vi "Channel Subpanel.vi"() -> ()   [LabVIEW 2021, in "CIF Manager UI.lvlib"]
uses:
  CIF Manager UI.lvlib
  CIFUI/Typedef/Channel Connection.ctl
  CIFUI/Typedef/Class Data for SubPanel.ctl
  <vilib>/gRPC/LabVIEW gRPC Library/Shared/grpcId.ctl
  CIFUI/Typedef/Core UI References.ctl
  CIFUI/Typedef/New Plugin.ctl
  CIFUI/Typedef/Run Listen Button.ctl
  CIFUI/Typedef/CIF_Manager_UI_Tab.ctl
  CIFUI/Typedef/SubPanel Events.ctl
  CIFUI/Typedef/New Connection Event Data.ctl
  CIFUI/Typedef/New Connection Plugin Event Data.ctl
  CIFUI/CIF_UI.lvclass
  CIFUI/CIF_UI.lvclass/CIF_UI.ctl
  CIFUI/Typedef/Direction to Include.ctl
  <vilib>/CIF Foundation/CIF Utilities/DataTypes/Typedef/Endian.ctl
  CIFUI/Typedef/Force Channel.ctl
  CIFUI/Utilities/Get Human Readable Error.vi
  <vilib>/CIF Foundation/CIF Utilities/Errors/Append Error Location.vi
  CIFUI/UI Element Update/Empty Tree by Reference.vi
  CIFUI/UI Element Update/Empty Table by Reference.vi
  CIFUI/UI Element Update/Initialize Manager Tab by Reference.vi
  <vilib>/CIF Foundation/CIF Utilities/Errors/Human Readable Error Message.vi
  <vilib>/CIF Foundation/CIF Utilities/DataTypes/DataTypes_CIF_U.lvlib
  <vilib>/gRPC/LabVIEW gRPC Library/grpc-lvsupport-release.lvlib
panel:
  in  "String Force":string
  in  "Class Data for SubPanel":T1
  in  "Force Active":bool
  in  "I64 Force":i64
  in  "U64 Force":u64
  in  "Double Force":dbl
  in  "Forced Data":string
  in  "Channel":string
  in  "Force Channel":bool
  in  "Link Channel":bool
  in  "Connection":T5
  in  "Publisher Channels":string(tree)
  in  "Subscriber Channels":string(tree)
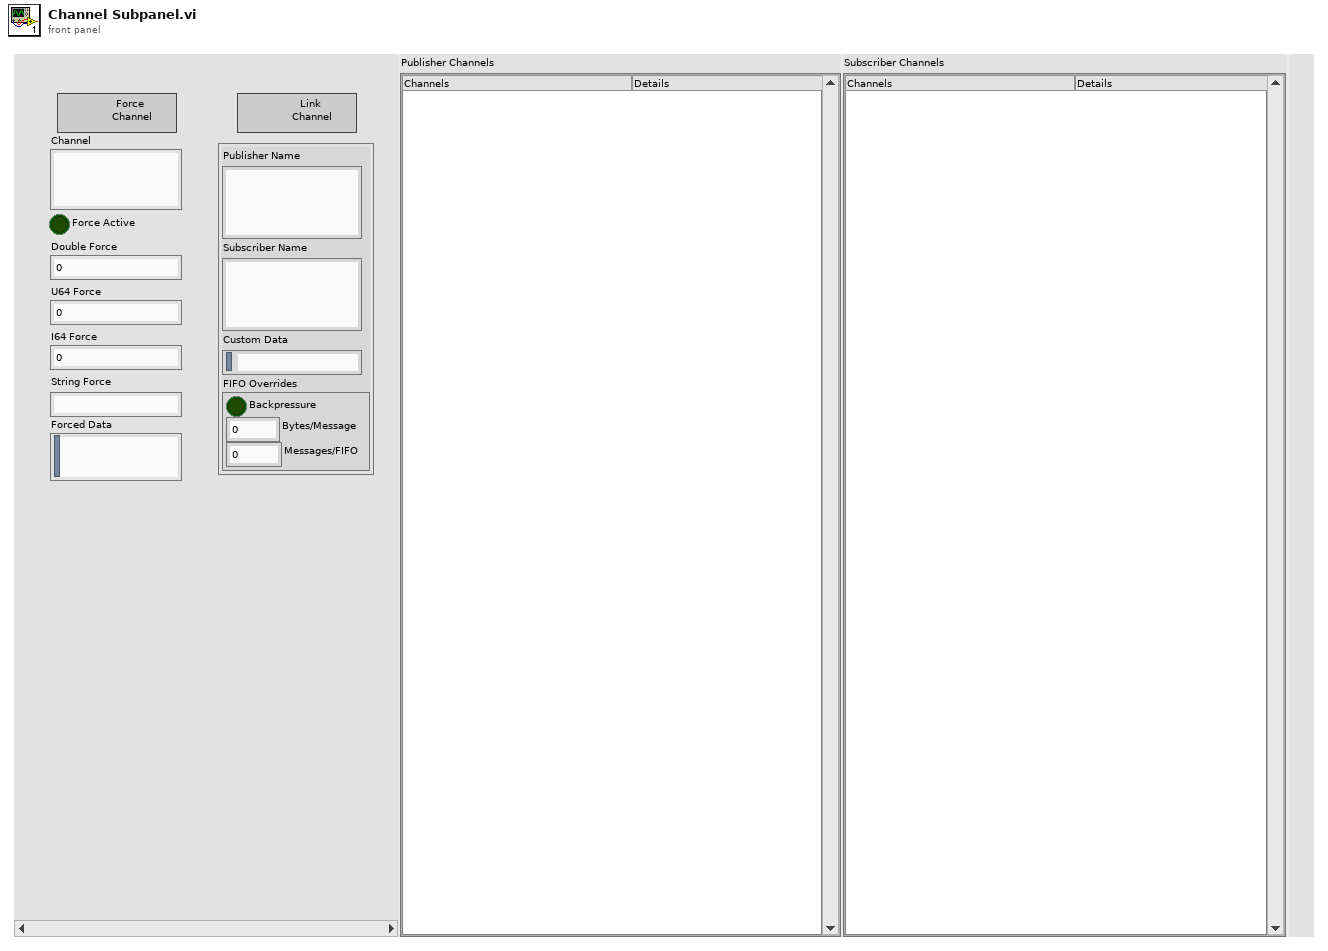
[diagram p1: front panel]
types:
  T1 = typedef "CIF_UI.lvclass/Class Data for SubPanel.ctl" = cluster{"IP Address":string, "Manager gRPC ID":T2, "Server Certificate File (.crt)":path, "Connected":bool, "Manager Connection":bool, "Core UI References":T3, "Subpanel Events":T4}
  T2 = typedef "grpc-lvsupport-release.lvlib/grpcId.ctl" = u64
  T3 = typedef "CIF_UI.lvclass/Core UI References.ctl" = cluster{"Discovered Plugins":refnum<vi>, "Discovered Plugins Valid":bool, "Loaded Plugins":refnum<vi>, "Loaded Plugins Valid":bool, "Publisher Channels":refnum<vi>, "Publisher Channels Valid":bool, "Subscriber Channels":refnum<vi>, "Subscriber Channels Valid":bool, "Plugin Status":refnum<vi>, "Plugin Status Valid":bool, "Channel Connection":refnum<vi>, "Channel Connection Valid":bool, "New Plugin Load":refnum<vi>, "New Plugin Load Valid":bool, "Errors":refnum<vi>, "Errors Valid":bool, "Plugin to Abort":refnum<vi>, "Plugin to Abort Valid":bool, "Connection":refnum<vi>, "Connection Valid":bool, "Exit":refnum<vi>, "Exit Valid":bool, "Run Listen":refnum<vi>, "Run Listen Valid":bool, "CIF Manager Tab":refnum<vi>, "Manger Tab Valid":bool, "Clear Local Error":refnum<vi>, "Clear Local Error Valid":bool, "Local Error":refnum<vi>, "Local Error Valid":bool, "System Errors":refnum<vi>, "System Errors Valid":bool, "Plugin Selection":refnum<vi>, "Plugin Selection Valid":bool}
  T4 = typedef "CIF_UI.lvclass/SubPanel Events.ctl" = cluster{"Clear Local Error":refnum<user-event>, "Shutdown":refnum<user-event>, "gRPC Connection":refnum<user-event>, "Plugin Connection":refnum<user-event>}
  T5 = typedef "CIF_UI.lvclass/Channel Connection.ctl" = cluster{"Publisher Name":string, "Subscriber Name":string, "Custom Data":string, "FIFO Overrides":cluster{"Backpressure":bool, "Bytes/Message":u32, "Messages/FIFO":u32}}
  T6 = typedef "CIF_UI.lvclass/Direction to Include.ctl" = enum16{"All", "Subscriber", "Publisher"}
  T7 = enum16{"big-endian, network order", "native, host order", "little-endian"}
  T8 = typedef "DataTypes_CIF_U.lvlib/Endian.ctl" = enum16{"Little Endian", "Big Endian"}
  T9 = typedef "CIF_UI.lvclass/Force Channel.ctl" = cluster{"channel_name":string, "force":bool, "force_data":string}
  T10 = typedef "CIFCoreChannel_client.lvlib/cif_management_common_Channel.ctl" = cluster{"name":string, "direction":T11, "type":string, "custom_config":u8[], "connected":bool, "connected_name":string, "forced":bool, "channel_pattern":T12}
  T11 = typedef "CIFCoreChannel_client.lvlib/cif_management_common_ChannelDirection.ctl" = enum32{"CHANNELDIRECTION_UNKNOWN", "CHANNELDIRECTION_PUBLISHER", "CHANNELDIRECTION_SUBSCRIBER"}
  T12 = typedef "CIFCoreChannel_client.lvlib/cif_management_common_ChannelPattern.ctl" = enum32{"CHANNELPATTERN_UNKNOWN", "CHANNELPATTERN_TAG", "CHANNELPATTERN_FIFO", "CHANNELPATTERN_MULTIFIFO", "CHANNELPATTERN_BACKPRESSUREFIFO"}
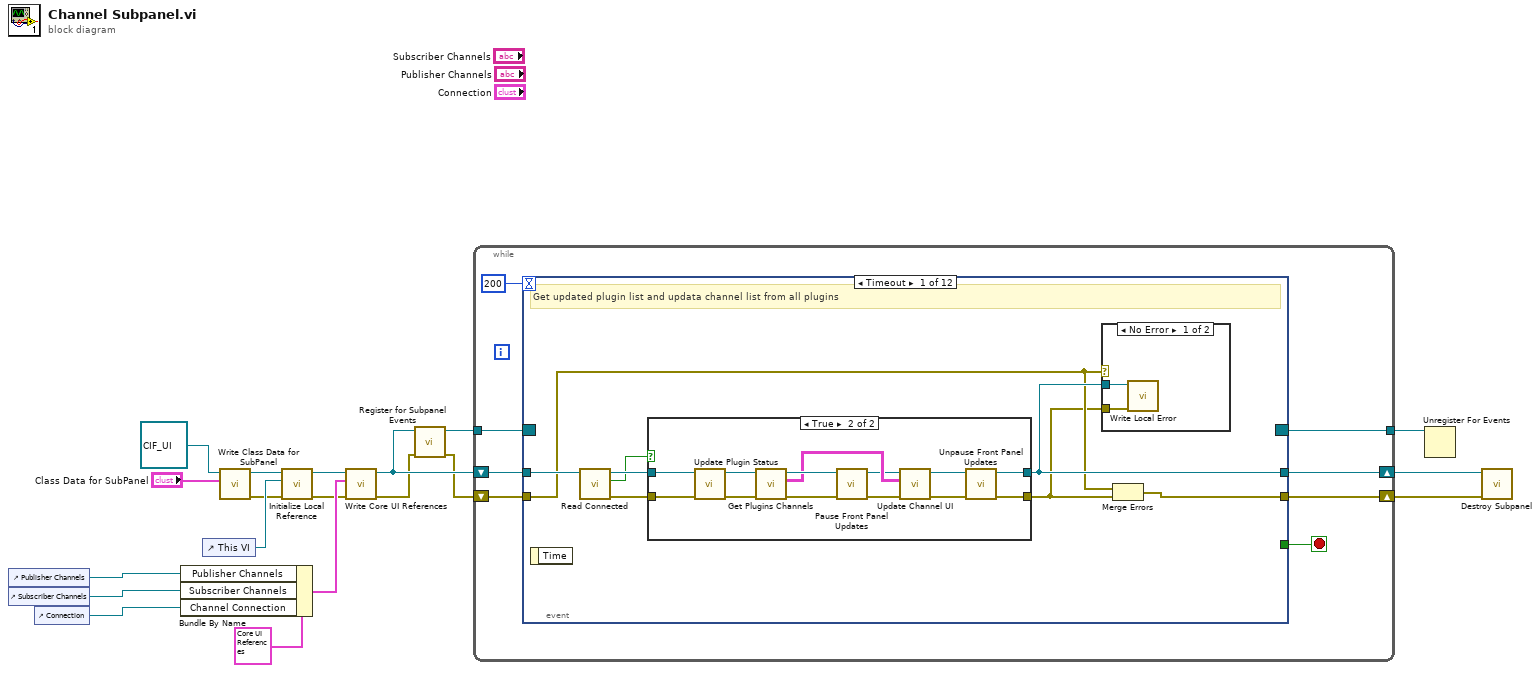
[diagram p0: block diagram]
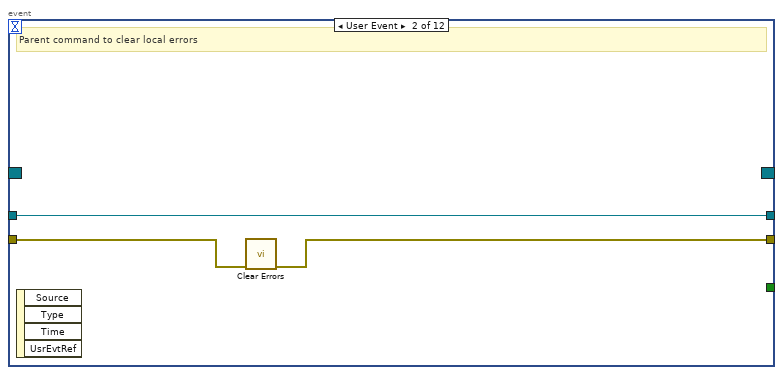
[diagram p4: hidden frame]
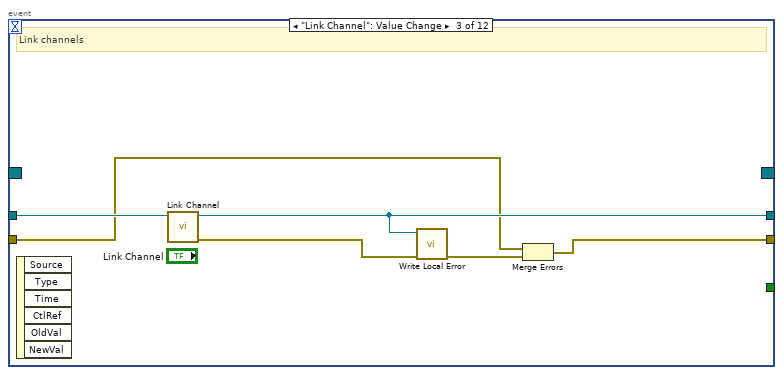
[diagram p5: hidden frame]
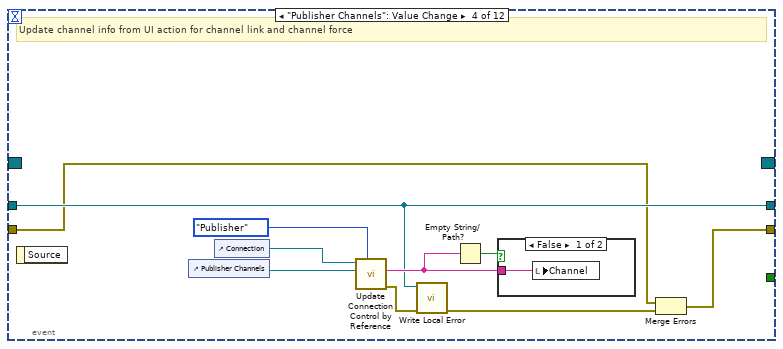
[diagram p6: hidden frame]
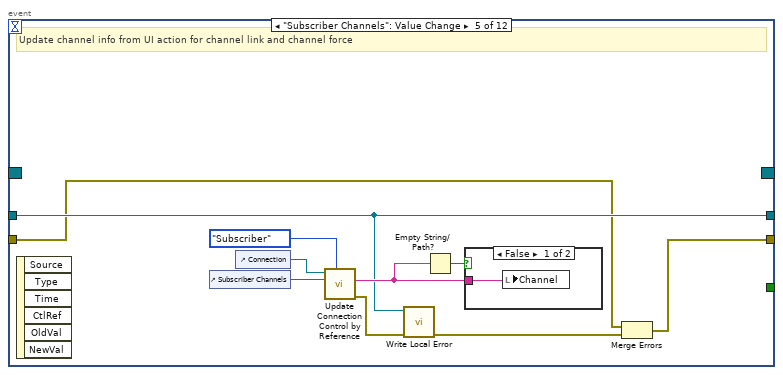
[diagram p8: hidden frame]
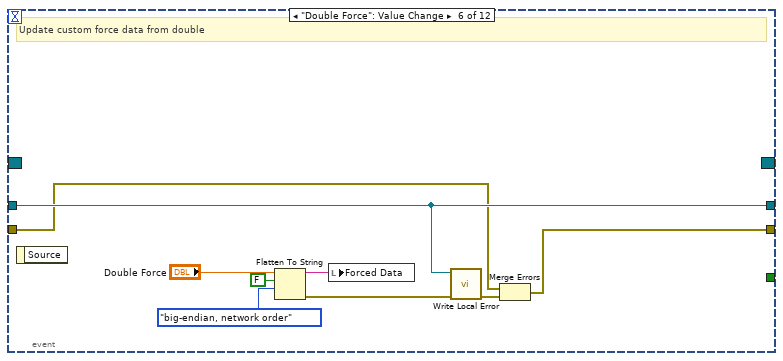
[diagram p10: hidden frame]
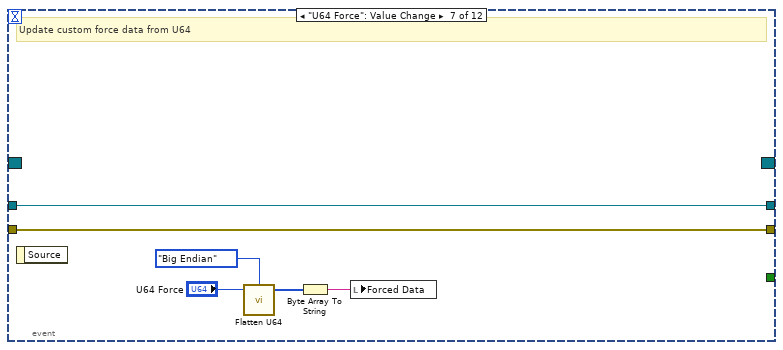
[diagram p11: hidden frame]
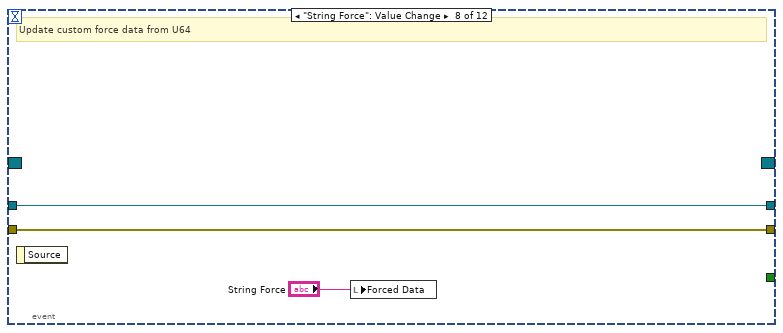
[diagram p12: hidden frame]
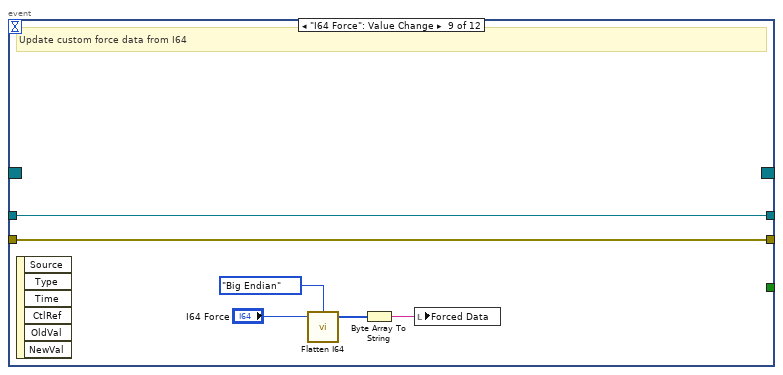
[diagram p13: hidden frame]
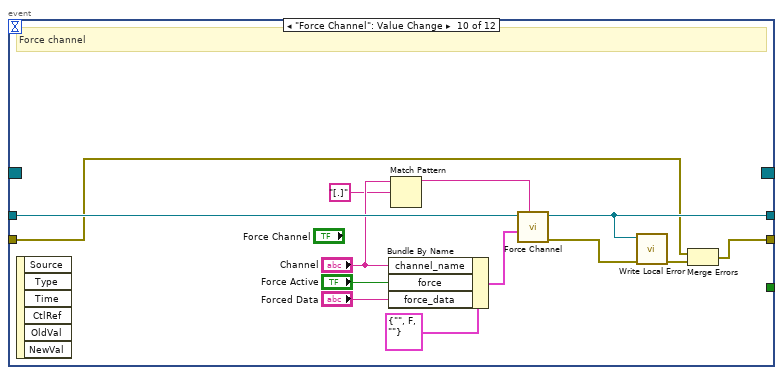
[diagram p14: hidden frame]
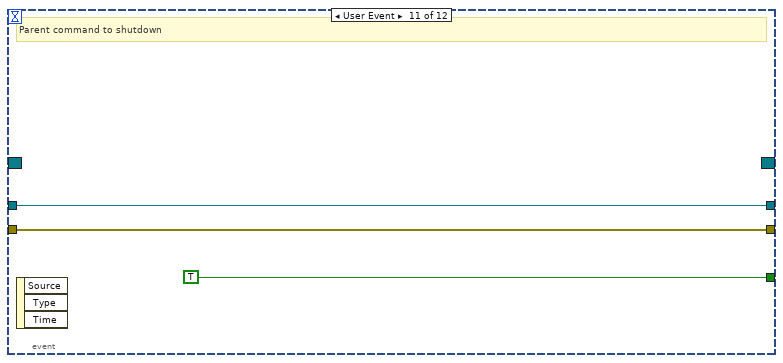
[diagram p15: hidden frame]
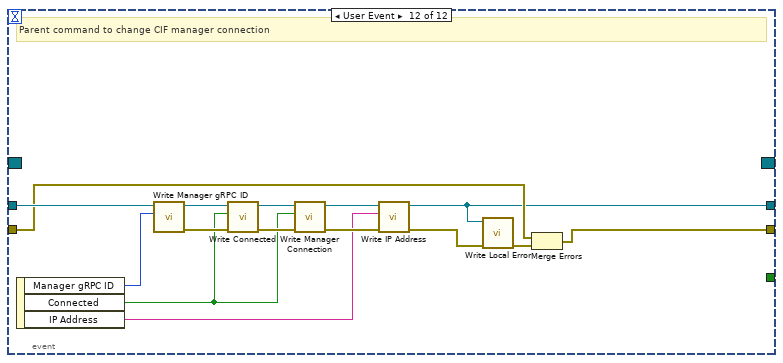
[diagram p16: hidden frame]
diagram:
  n1 = control-ref of="Publisher Channels"() -> (w19:refnum<vi>)
  n2 = control-ref of="Subscriber Channels"() -> (w18:refnum<vi>)
  n3 = control-ref of="Connection"() -> (w17:refnum<vi>)
  n4 = Bundle By Name(cluster=T3 {"Discovered Plugins"=refnum, "Discovered Plugins Valid"=FALSE, "Loaded Plugins"=refnum, "Loaded Plugins Valid"=FALSE, "Publisher Channels"=refnum, "Publisher Channels Valid"=FALSE, "Subscriber Channels"=refnum, "Subscriber Channels Valid"=FALSE, "Plugin Status"=refnum, "Plugin Status Valid"=FALSE, "Channel Connection"=refnum, "Channel Connection Valid"=FALSE, "New Plugin Load"=refnum, "New Plugin Load Valid"=FALSE, "Errors"=refnum, "Errors Valid"=FALSE, "Plugin to Abort"=refnum, "Plugin to Abort Valid"=FALSE, "Connection"=refnum, "Connection Valid"=FALSE, "Exit"=refnum, "Exit Valid"=FALSE, "Run Listen"=refnum, "Run Listen Valid"=FALSE, "CIF Manager Tab"=refnum, "Manger Tab Valid"=FALSE, "Clear Local Error"=refnum, "Clear Local Error Valid"=FALSE, "Local Error"=refnum, "Local Error Valid"=FALSE, "System Errors"=refnum, "System Errors Valid"=FALSE, "Plugin Selection"=refnum, "Plugin Selection Valid"=FALSE} ("UI References"), "Publisher Channels"=w19, "Subscriber Channels"=w18, "Channel Connection"=w17) -> (w15:T3)
  n5 = control-ref of="This VI"() -> (w10:refnum<vi>)
  n6 = call "Write Class Data for SubPanel.vi"("Class Data for SubPanel"="Class Data for SubPanel", "CIF_UI in"=refnum<class "CIF_UI.lvclass"> refnum) -> ("error out"=w3:errorcluster, "CIF_UI out"=w4:refnum<class "CIF_UI.lvclass">)  [unwired: 8 in]
  n7 = call "Initialize Local Reference.vi"("error in (no error)"=w3, "This VI"=w10, "CIF_UI in"=w4) -> ("error out"=w8:errorcluster, "CIF_UI out"=w9:refnum<class "CIF_UI.lvclass">)  [unwired: 7 in]
  n8 = call "Write Core UI References.vi"("error in (no error)"=w8, "UI References"=w15, "CIF_UI in"=w9) -> ("error out"=w12:errorcluster, "CIF_UI out"=w14:refnum<class "CIF_UI.lvclass">)  [unwired: 7 in]
  n9 = call "Register for Subpanel Events.vi"("error in (no error)"=w12, "CIF_UI in"=w14) -> ("error out"=w11:errorcluster, "Event Registration Refnum"=w13:refnum<event-registration>)  [unwired: 8 in]
  n10 = while {
    tunnel: w13 -> [w26]
    shift-right: [w22] -> w7
    shift-left: w14 -> [w24]
    shift-right: [w20] -> w1
    shift-left: w11 -> [w23]
    tunnel: [w21] -> w2
    stop <- w25 stop-if-true
    n11 = event shown="[0] Timeout" {
      selector: w26 -> [_ _ _ _ _ _ _ _ _ _ _ _]
      dyn-events: [_ _ _ _ _ _ _ _ _ _ _ _] -> w21
      timeout: 200 -> [_ _ _ _ _ _ _ _ _ _ _ _]
      tunnel: [_ _ _ _ _ _ _ _ _ _ TRUE _] -> w25
      tunnel: w24 -> [w32 w53 w61 w65 w76 w86 w98 w101 w103 w120 w122 w132]
      tunnel: w23 -> [w30 w55 w57 w63 w73 w85 w97 w100 w102 w108 w121 w125]
      tunnel: [w28 w54 w56 w62 w74 w84 w97 w100 w102 w109 w121 w126] -> w20
      tunnel: [w31 w53 w60 w65 w76 w86 w98 w101 w103 w112 w122 w124] -> w22
      event Timeout {
        # "Get updated plugin list and updata channel list from all plugins"
        n12 = event-data() -> ()  [unwired: 1 in, 1 out]
        n13 = call "Read Connected.vi"("CIF_UI in"=w32) -> ("error out"=w34:errorcluster, "Connected"=w33:bool, "CIF_UI out"=w35:refnum<class "CIF_UI.lvclass">)  [unwired: 8 in]
        n14 = case shown="True" w33 {
          tunnel: w34 -> [w38 w45]
          tunnel: [w38 w52] -> w29
          tunnel: w35 -> [w39 w46]
          tunnel: [w39 w51] -> w31
          frame False {
          }
          frame True {
            n15 = call "Update Plugin Status.vi"("error in (no error)"=w45, "CIF_UI in"=w46) -> ("error out"=w49:errorcluster, "CIF_UI out"=w50:refnum<class "CIF_UI.lvclass">)  [unwired: 8 in]
            n16 = call "Get Plugins Channels.vi"("error in (no error)"=w49, "CIF_UI in"=w50) -> ("error out"=w41:errorcluster, "Channels"=w43:T10[][], "CIF_UI out"=w44:refnum<class "CIF_UI.lvclass">)  [unwired: 6 in, 1 out]
            n17 = call "Pause Front Panel Updates.vi"("error in (no error)"=w41, "CIF_UI in"=w44) -> ("error out"=w40:errorcluster, "CIF_UI out"=w42:refnum<class "CIF_UI.lvclass">)  [unwired: 8 in]
            n18 = call "Update Channel UI.vi"("error in (no error)"=w40, "Channels"=w43, "CIF_UI in"=w42) -> ("error out"=w47:errorcluster, "CIF_UI out"=w48:refnum<class "CIF_UI.lvclass">)  [unwired: 7 in]
            n19 = call "Unpause Front Panel Updates.vi"("error in (no error)"=w47, "CIF_UI in"=w48) -> ("error out"=w52:errorcluster, "CIF_UI out"=w51:refnum<class "CIF_UI.lvclass">)  [unwired: 8 in]
          }
        }
        n20 = case shown="No Error" w30 {
          tunnel: w29 -> [w37 _]
          tunnel: w31 -> [w36 _]
          frame No Error {
            n21 = call "Write Local Error.vi"("error in (no error)"=w37, "CIF_UI in"=w36) -> ()  [unwired: 9 in, 1 out]
          }
          frame Error {
          }
        }
        n22 = Merge Errors(w30, w29) -> (w28:errorcluster)
      }
      event User Event {
        # "Parent command to clear local errors"
        n23 = event-data() -> ()  [unwired: 1 in, 4 out]
        n24 = call <vilib>:"Clear Errors.vi"("error in (no error)"=w55) -> ("error out"=w54:errorcluster)  [unwired: 5 in, 1 out]
      }
      event "Link Channel": Value Change {
        # "Link channels"
        n25 = event-data() -> ()  [unwired: 1 in, 6 out]
        n26 = call "Link Channel.vi"("CIF_UI in"=w61) -> ("error out"=w59:errorcluster, "CIF_UI out"=w60:refnum<class "CIF_UI.lvclass">)  [unwired: 9 in]
        n27 = call "Write Local Error.vi"("error in (no error)"=w59, "CIF_UI in"=w60) -> ("error out"=w58:errorcluster)  [unwired: 9 in]
        n28 = Merge Errors(w57, w58) -> (w56:errorcluster)
      }
      event "Publisher Channels": Value Change {
        # "Update channel info from UI action for channel link and channel force"
        n29 = event-data() -> ()  [unwired: 1 in, 1 out]
        n30 = control-ref of="Publisher Channels"() -> (w69:refnum<vi>)
        n31 = control-ref of="Connection"() -> (w70:refnum<vi>)
        n32 = call "Update Connection Control by Reference.vi"("Direction to Include"=Direction_to_Include."Publisher", "Channels"=w69, "Channel Connection"=w70) -> ("error out"=w66:errorcluster, "Channel Name"=w67:string)  [unwired: 7 in]
        n33 = call "Write Local Error.vi"("error in (no error)"=w66, "CIF_UI in"=w65) -> ("error out"=w64:errorcluster)  [unwired: 9 in]
        n34 = Empty String/Path?(string/path=w67) -> (empty?=w68:bool)
        n35 = case shown="False" w68 {
          tunnel: w67 -> [w72 _]
          frame False {
            n36 = local write "Channel"(w72) -> ()
          }
          frame True {
          }
        }
        n37 = Merge Errors(w63, w64) -> (w62:errorcluster)
      }
      event "Subscriber Channels": Value Change {
        # "Update channel info from UI action for channel link and channel force"
        n38 = event-data() -> ()  [unwired: 1 in, 6 out]
        n39 = control-ref of="Subscriber Channels"() -> (w80:refnum<vi>)
        n40 = control-ref of="Connection"() -> (w81:refnum<vi>)
        n41 = call "Update Connection Control by Reference.vi"("Direction to Include"=Direction_to_Include."Subscriber", "Channels"=w80, "Channel Connection"=w81) -> ("error out"=w77:errorcluster, "Channel Name"=w78:string)  [unwired: 7 in]
        n42 = call "Write Local Error.vi"("error in (no error)"=w77, "CIF_UI in"=w76) -> ("error out"=w75:errorcluster)  [unwired: 9 in]
        n43 = Empty String/Path?(string/path=w78) -> (empty?=w79:bool)
        n44 = case shown="False" w79 {
          tunnel: w78 -> [w83 _]
          frame False {
            n45 = local write "Channel"(w83) -> ()
          }
          frame True {
          }
        }
        n46 = Merge Errors(w73, w75) -> (w74:errorcluster)
      }
      event "Double Force": Value Change {
        # "Update custom force data from double"
        n47 = event-data() -> ()  [unwired: 1 in, 1 out]
        n48 = Flatten To String(anything="Double Force", prepend array or string size? (T)=FALSE, byte order (0:big-endian, network order)=T7."big-endian, network order") -> (data string=w89:string, error out=w87:errorcluster)  [unwired: 1 in, 1 out]
        n49 = local write "Forced Data"(w89) -> ()
        n50 = call "Write Local Error.vi"("error in (no error)"=w87, "CIF_UI in"=w86) -> ("error out"=w88:errorcluster)  [unwired: 9 in]
        n51 = Merge Errors(w85, w88) -> (w84:errorcluster)
      }
      event "U64 Force": Value Change {
        # "Update custom force data from U64"
        n52 = event-data() -> ()  [unwired: 1 in, 1 out]
        n53 = call <vilib>:"Flatten U64.vi"("U64"="U64 Force", "Endian"=Endian."Big Endian") -> ("Flat Data"=w94:u8[])  [unwired: 3 in]
        n54 = Byte Array To String(unsigned byte array=w94) -> (string=w95:string)
        n55 = local write "Forced Data"(w95) -> ()
      }
      event "String Force": Value Change {
        # "Update custom force data from U64"
        n56 = event-data() -> ()  [unwired: 1 in, 1 out]
        n57 = local write "Forced Data"("String Force") -> ()
      }
      event "I64 Force": Value Change {
        # "Update custom force data from I64"
        n58 = event-data() -> ()  [unwired: 1 in, 6 out]
        n59 = call <vilib>:"Flatten I64.vi"("I64"="I64 Force", "Endian"=Endian."Big Endian") -> ("Flat Data"=w106:u8[])  [unwired: 3 in]
        n60 = Byte Array To String(unsigned byte array=w106) -> (string=w107:string)
        n61 = local write "Forced Data"(w107) -> ()
      }
      event "Force Channel": Value Change {
        # "Force channel"
        n62 = event-data() -> ()  [unwired: 1 in, 6 out]
        n63 = Bundle By Name(cluster=T9 {"channel_name"="", "force"=FALSE, "force_data"=""} ("Force Channel"), "channel_name"="Channel", "force"="Force Active", "force_data"="Forced Data") -> (w118:T9)
        n64 = Match Pattern(string="Channel", regular expression="[.]") -> (before substring=w113:string)  [unwired: 1 in, 3 out]
        n65 = call "Force Channel.vi"("Plugin Name"=w113, "Force Channel"=w118, "CIF_Plugin_UI in"=w120) -> ("error out"=w111:errorcluster, "CIF_Plugin_UI out"=w112:refnum<class "CIF_UI.lvclass">)  [unwired: 6 in, 1 out]
        n66 = call "Write Local Error.vi"("error in (no error)"=w111, "CIF_UI in"=w112) -> ("error out"=w110:errorcluster)  [unwired: 9 in]
        n67 = Merge Errors(w108, w110) -> (w109:errorcluster)
      }
      event User Event {
        # "Parent command to shutdown"
        n68 = event-data() -> ()  [unwired: 1 in, 3 out]
      }
      event User Event {
        # "Parent command to change CIF manager connection"
        n69 = event-data() -> ("Manager gRPC ID"=w129:T2, "Connected"=w130:bool, "IP Address"=w131:string)  [unwired: 1 in]
        n70 = call "Write Manager gRPC ID.vi"("gRPCid"=w129, "CIF_UI in"=w132) -> ("error out"=w134:errorcluster, "CIF_UI out"=w133:refnum<class "CIF_UI.lvclass">)  [unwired: 8 in]
        n71 = call "Write Connected.vi"("error in (no error)"=w134, "Connected"=w130, "CIF_UI in"=w133) -> ("error out"=w136:errorcluster, "CIF_UI out"=w135:refnum<class "CIF_UI.lvclass">)  [unwired: 7 in]
        n72 = call "Write Manager Connection.vi"("error in (no error)"=w136, "Manager Connection"=w130, "CIF_UI in"=w135) -> ("error out"=w138:errorcluster, "CIF_UI out"=w137:refnum<class "CIF_UI.lvclass">)  [unwired: 7 in]
        n73 = call "Write IP Address.vi"("error in (no error)"=w138, "IP Address"=w131, "CIF_UI in"=w137) -> ("error out"=w127:errorcluster, "CIF_UI out"=w124:refnum<class "CIF_UI.lvclass">)  [unwired: 7 in]
        n74 = call "Write Local Error.vi"("error in (no error)"=w127, "CIF_UI in"=w124) -> ("error out"=w128:errorcluster)  [unwired: 9 in]
        n75 = Merge Errors(w125, w128) -> (w126:errorcluster)
      }
    }
  }
  n76 = Unregister For Events(event registration refnum=w2) -> ()  [unwired: 1 in, 1 out]
  n77 = call "Destroy Subpanel.vi"("error in (no error)"=w1, "CIF_UI in"=w7) -> ()  [unwired: 8 in, 2 out]
